vi "hist_search.vi"(8 "ave_m":dbl, 9 "ave_t":dbl, 10 "model":dbl[](array[numeric]), 11 "target":dbl[](array[numeric])) -> (0 "error":dbl, 3 "displacement":dbl)   [LabVIEW 2012]
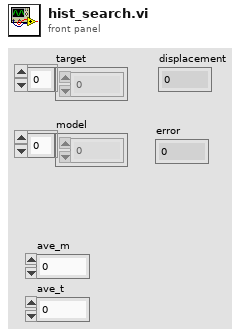
[diagram p1: front panel]
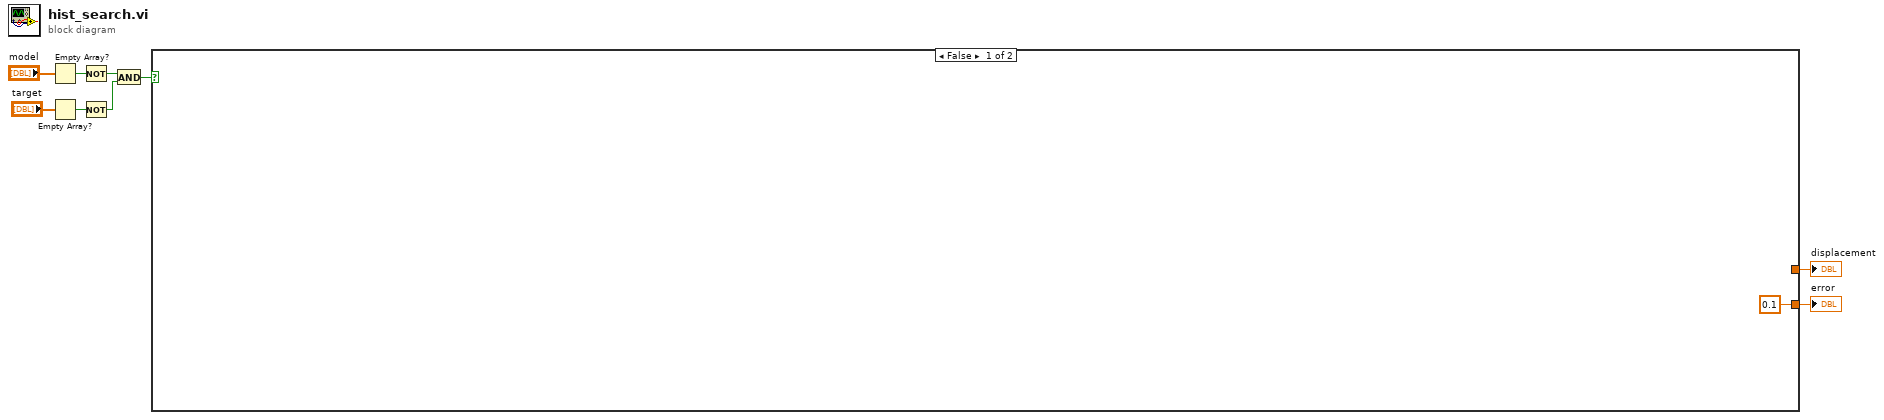
[diagram p0: block diagram]
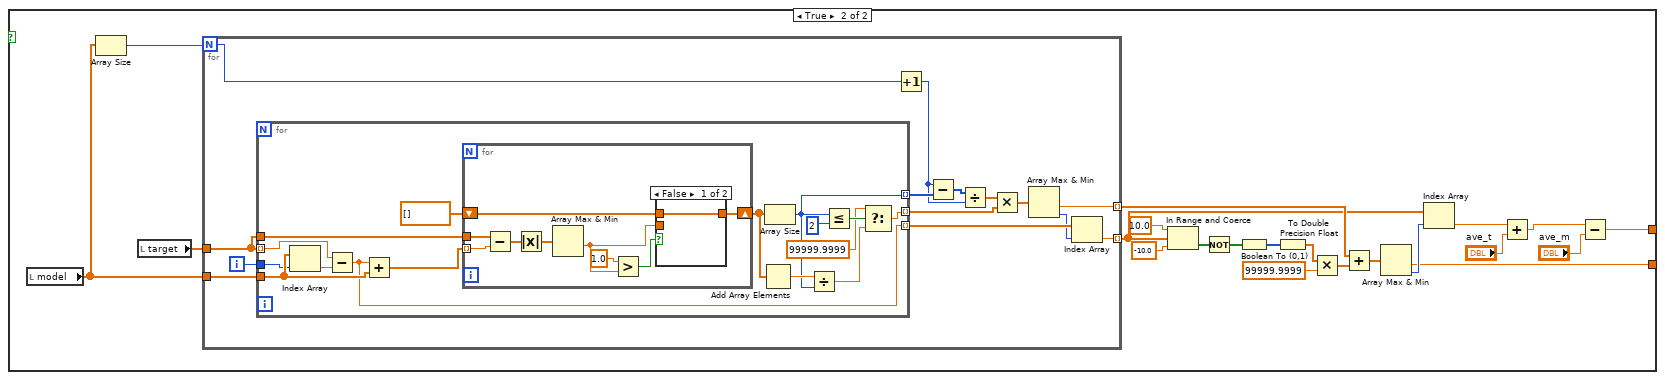
[diagram p2: hidden frame]
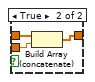
[diagram p3: hidden frame]
diagram:
  n1 = Empty Array?(array="model") -> (empty?=w5:bool)
  n2 = Empty Array?(array="target") -> (empty?=w4:bool)
  n3 = Not(x=w5) -> (.not. x?=w3:bool)
  n4 = Not(x=w4) -> (.not. x?=w2:bool)
  n5 = And(x=w3, y=w2) -> (x .and. y?=w1:bool)
  n6 = case shown="False" w1 {
    tunnel: [0.1 w18] -> w9
    tunnel: [_ w13] -> w8
    frame False {
    }
    frame True {
      n7 = local read "model"() -> (w12:dbl[])
      n8 = Array Size(array=w12) -> (size(s)=w19:i32)
      n9 = local read "target"() -> (w11:dbl[])
      n10 = for {
        N: w19 -> [w33]
        tunnel: w12 -> [w45]
        tunnel: [w38] -> w21 mode=indexing
        tunnel: [w37] -> w29 mode=indexing
        tunnel: w11 -> [w36]
        i -> [w43]
        n11 = for {
          tunnel: w36 -> [w61]
          tunnel: w45 -> [w58]
          tunnel: [w49] -> w35 mode=indexing
          tunnel: [w53] -> w42 mode=indexing
          tunnel: [w55] -> w40 mode=indexing
          tunnel: w36 -> [w56] mode=indexing
          tunnel: w43 -> [w54]
          n12 = Index Array(array=w58, index=w54) -> (element=w57:dbl)
          n13 = Subtract(x=w56, y=w57) -> (x-y=w55:dbl)
          n14 = Add(x=w55, y=w58) -> (x+y=w59:dbl[])
          n15 = for {
            tunnel: w61 -> [w70]
            tunnel: w59 -> [w69] mode=indexing
            shift-right: [w63] -> w47
            shift-left: dbl[] [] -> [w62]
            n16 = Subtract(x=w70, y=w69) -> (x-y=w68:dbl[])
            n17 = Absolute Value(x=w68) -> (abs(x)=w67:dbl[])
            n18 = Array Max & Min(array=w67) -> (min value=w64:dbl)  [unwired: 3 out]
            n19 = Greater?(x=1.0, y=w64) -> (0:w65:bool)
            n20 = case shown="False" w65 {
              tunnel: w64 -> [_ w74]
              tunnel: [w71 w73] -> w63
              tunnel: w62 -> [w71 w72]
              frame False {
              }
              frame True {
                n21 = Build Array (concatenate)(w72, w74) -> (w73:dbl[])
              }
            }
          }
          n22 = Add Array Elements(numeric array=w47) -> (sum=w60:dbl)
          n23 = Array Size(array=w47) -> (size(s)=w53:i32)
          n24 = Divide(x=w60, y=w53) -> (x/y=w50:dbl)
          n25 = Less Or Equal?(x=w53, y=2) -> (x <= y?=w51:bool)
          n26 = Select(t=99999.9999, s=w51, f=w50) -> (s? t:f=w49:dbl)
        }
        n27 = Increment(x=w33) -> (x+1=w32:i32)
        n28 = Subtract(x=w32, y=w42) -> (x-y=w44:i32[])
        n29 = Divide(x=w44, y=w32) -> (x/y=w34:dbl[])
        n30 = Multiply(x=w34, y=w35) -> (x*y=w41:dbl[])
        n31 = Array Max & Min(array=w41) -> (min value=w37:dbl, min index (indices)=w39:i32)  [unwired: 2 out]
        n32 = Index Array(array=w40, index=w39) -> (element=w38:dbl)
      }
      n33 = In Range and Coerce(upper limit=10.0, x=w21, lower limit=-10.0) -> (In Range?=w24:bool[])  [unwired: 1 out]
      n34 = Not(x=w24) -> (.not. x?=w25:bool[])
      n35 = Boolean To (0,1)(Boolean=w25) -> (0, 1=w26:i16[])
      n36 = To Double Precision Float(number=w26) -> (double precision float=w27:dbl[])
      n37 = Multiply(x=w27, y=99999.9999) -> (x*y=w28:dbl[])
      n38 = Add(x=w29, y=w28) -> (x+y=w30:dbl[])
      n39 = Array Max & Min(array=w30) -> (min value=w18:dbl, min index (indices)=w20:i32)  [unwired: 2 out]
      n40 = Index Array(array=w21, index=w20) -> (element=w17:dbl)
      n41 = Add(x=w17, y="ave_t") -> (x+y=w15:dbl)
      n42 = Subtract(x=w15, y="ave_m") -> (x-y=w13:dbl)
    }
  }
  "displacement" <- w8
  "error" <- w9
